vi "Browser Print Format.vi"(3 "error in (no error)":errorcluster, 5 "Format":T1={"header"="default", "footer"="default", "margin_bottom"="default", "margin_left"="default", "margin_right"="default", "margin_top"="default"}) -> (0 "error out":errorcluster, 2 "Previous Values":T1={"header"="default", "footer"="default", "margin_bottom"="default", "margin_left"="default", "margin_right"="default", "margin_top"="default"})   [LabVIEW 2019]
doc: "This VI can be used to set print formatting options when using the Microsoft Internet Browser or Web Browser Control. It can set the header footer and margins. It cannot set the orientation. Orientation can be set in the defualt printer settings.\n\nIf you do not want to change one of the values, leave it \"default\".\n\n*Warning - This VI sets the printer setting registry entries and will change the settings for all instances of the browser. The previous values will be returned from the VI so that they can be restored later if desired.\n\nFormat Cluster:\n0) header\n1) footer\n2) margin_bottom\n3) margin_left\n4) margin_right\n5) margin_top"
uses:
  <vilib>/registry/registry.llb/Registry RtKey.ctl
  <vilib>/registry/registry.llb/Write Registry Value Simple STR.vi
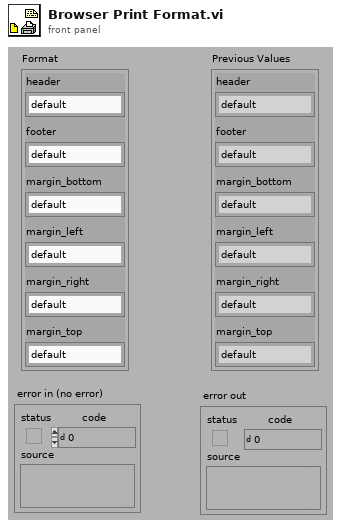
[diagram p1: front panel]
types:
  T1 = cluster{"header":string, "footer":string, "margin_bottom":string, "margin_left":string, "margin_right":string, "margin_top":string}
  T2 = enum32{"KEY_QUERY_VALUE", "KEY_SET_VALUE", "KEY_CREATE_SUB_KEY", "KEY_ENUMERATE_SUB_KEYS", "KEY_NOTIFY", "KEY_CREATE_LINK", "KEY_READ", "KEY_WRITE", "KEY_ALL_ACCESS", "KEY_READ | KEY_WRITE"}
  T3 = typedef "Registry RtKey.ctl" = enum32{"HKEY_CLASSES_ROOT", "HKEY_CURRENT_USER", "HKEY_LOCAL_MACHINE", "HKEY_USERS", "HKEY_PERFORMANCE_DATA", "HKEY_CURRENT_CONFIG", "HKEY_DYN_DATA"}
  T4 = typedef "Registry refnum.ctl" = refnum<k1>
  T5 = cluster{"numValues":i32, "maxValueNameLen":i32, "maxValueDataLen":i32}
  T6 = cluster{"String/Binary data[0]":string, "String/Binary data[1]":string, "String/Binary data[2]":string, "String/Binary data[3]":string, "String/Binary data[4]":string, "String/Binary data[5]":string}
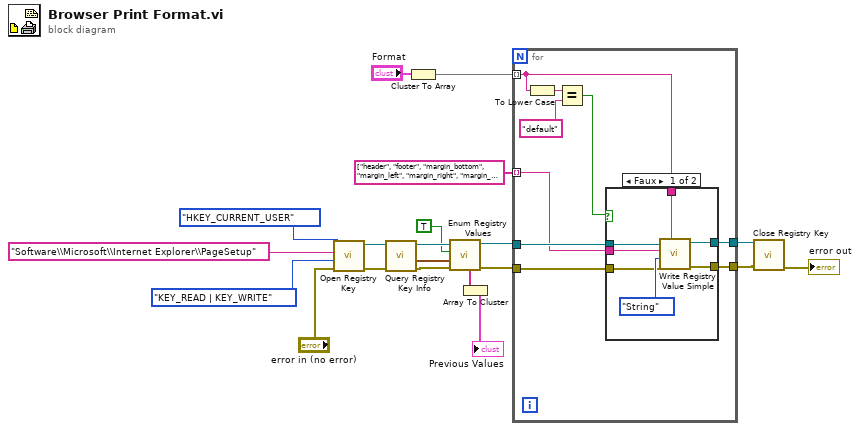
[diagram p0: block diagram]
diagram:
  n1 = call <vilib>:"Open Registry Key.vi"("error in (no error)"="error in (no error)", "security access mask (KEY_READ | KEY_WRITE)"=T2."KEY_READ | KEY_WRITE", "subkey"="Software\\Microsoft\\Internet Explorer\\PageSetup", "root key (HKEY_LOCAL_MACHINE)"=Registry_RtKey."HKEY_CURRENT_USER") -> ("error out"=w8:errorcluster, "refnum out"=w7:T4)  [unwired: 6 in]
  n2 = call <vilib>:"Query Registry Key Info.vi"("error in (no error)"=w8, "refnum"=w7) -> ("error out"=w9:errorcluster, "value info"=w3:T5, "refnum out"=w6:T4)  [unwired: 5 in, 2 out]
  n3 = Cluster To Array(cluster="Format") -> (array=w13:string[])
  n4 = call <vilib>:"Enum Registry Values.vi"("error in (no error)"=w9, "value info"=w3, "retrieve data? (F)"=TRUE, "refnum"=w6) -> ("error out"=w10:errorcluster, "refnum out"=w4:T4, "String/Binary data"=w2:string[])  [unwired: 2 in, 3 out]
  n5 = Array To Cluster(array=w2) -> (cluster=→"Previous Values":T6)
  n6 = for {
    tunnel: [w29] -> w17
    tunnel: [w28] -> w16
    tunnel: w13 -> [w25] mode=indexing
    tunnel: w4 -> [w23]
    tunnel: w10 -> [w22]
    tunnel: string[] ["header", "footer", "margin_bottom", "margin_left", "margin_right", "margin_top"] ("values") -> [w21] mode=indexing
    n7 = To Lower Case(string=w25) -> (all lower case string=w27:string)
    n8 = Equal?(x=w27, y="default") -> (x = y?=w24:bool)
    n9 = case shown="Faux" w24 {
      tunnel: [w36 w37] -> w29
      tunnel: [w35 w38] -> w28
      tunnel: w25 -> [w33 _]
      tunnel: w23 -> [w32 w38]
      tunnel: w22 -> [w31 w37]
      tunnel: w21 -> [w30 _]
      frame False {
        n10 = call-poly <vilib>:"Write Registry Value Simple.vi"("String/Binary data"=w33, "error in (no error)"=w31, "simple data type"=enum16{"String", "Binary", "DWORD"}."String", "value"=w30, "refnum"=w32) -> ("error out"=w36:errorcluster, "refnum out"=w35:T4)  [unwired: 3 in]
      }
      frame True {
      }
    }
  }
  n11 = call <vilib>:"Close Registry Key.vi"("error in (no error)"=w17, "refnum"=w16) -> ("error out"=→"error out":errorcluster)  [unwired: 5 in]
